vi "Flatten.vi"(8 "error in":errorcluster, 9 "Data":T1) -> (0 "error out":errorcluster, 2 "Buffer":u8[](array[numeric]) format="%.0x")   [LabVIEW 2020, in "CmdDigital.lvlib"]
uses:
  CmdDigital.lvlib
  Data.ctl
  lv-protoc/LV-Proto/LV-Proto.lvlib
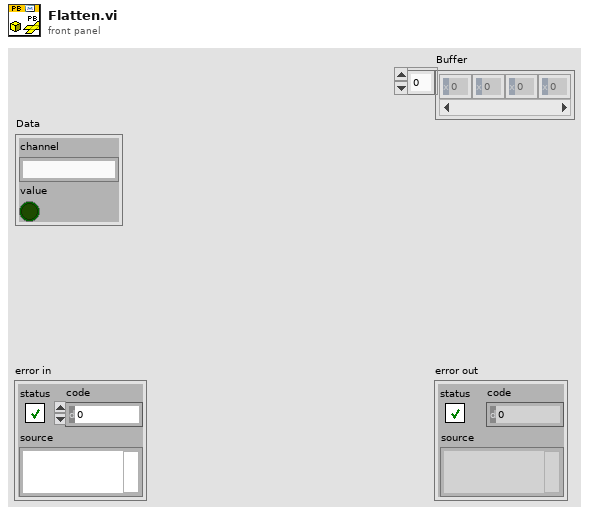
[diagram p1: front panel]
types:
  T1 = typedef "CmdDigital.lvlib/Data.ctl" = cluster{"channel":string, "value":bool}
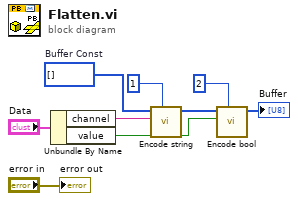
[diagram p0: block diagram]
diagram:
  w7 = u8[] []  # Buffer Const
  n1 = Unbundle By Name("Data") -> ("channel"=w5:string, "value"=w2:bool)
  n2 = call "Encode string.vi"("Field Number"=1, "string"=w5, "Buffer in"=w7) -> ("Buffer"=w4:u8[])  [unwired: 8 in]
  n3 = call "Encode bool.vi"("Field Number"=2, "Bool"=w2, "Buffer in"=w4) -> ("Buffer"=→"Buffer":u8[])  [unwired: 8 in]
  "error out" <- "error in"
